vi "CTL_Level SpecV2.vi"(6 "Index(n-1) In":i32[](array[numeric]), 7 "Full Config 2":T1, 8 "error in (no error)":errorcluster, 9 "Level IN inches":dbl=8.853199052567236, 10 "Index B":i32=3, 11 "Index A":i32=3) -> (0 "error out":errorcluster, 2 "Enable":bool, 3 "Specs Out":T5, 4 "Index(n-1) Out":i32[](array[numeric]))   [LabVIEW 2024]
doc: "Determine the row index and Specification from the Config File Spec Table for the given level. \nAlso detemines the flag state for these Flags:\n Switch Zone = Resitor switch levels must occur in this zone\n R In Range Zone = Resistor value must be specified level\n R measure = When to take the measurement to record."
uses:
  Control Definitions/DEF_SpecsOut.ctl
  Control Definitions/Def PumpCtlRefs.ctl
  Control Definitions/Def FullCfg.ctl
  Control Definitions/Def BenchCfg.ctl
  Control Definitions/Def Bench Status.ctl
  Control Definitions/Ded LUT_Status.ctl
  Control Definitions/Ded Spec RNG.ctl
panel:
  out "Index(n)":i32
  out "Boolean":bool=TRUE
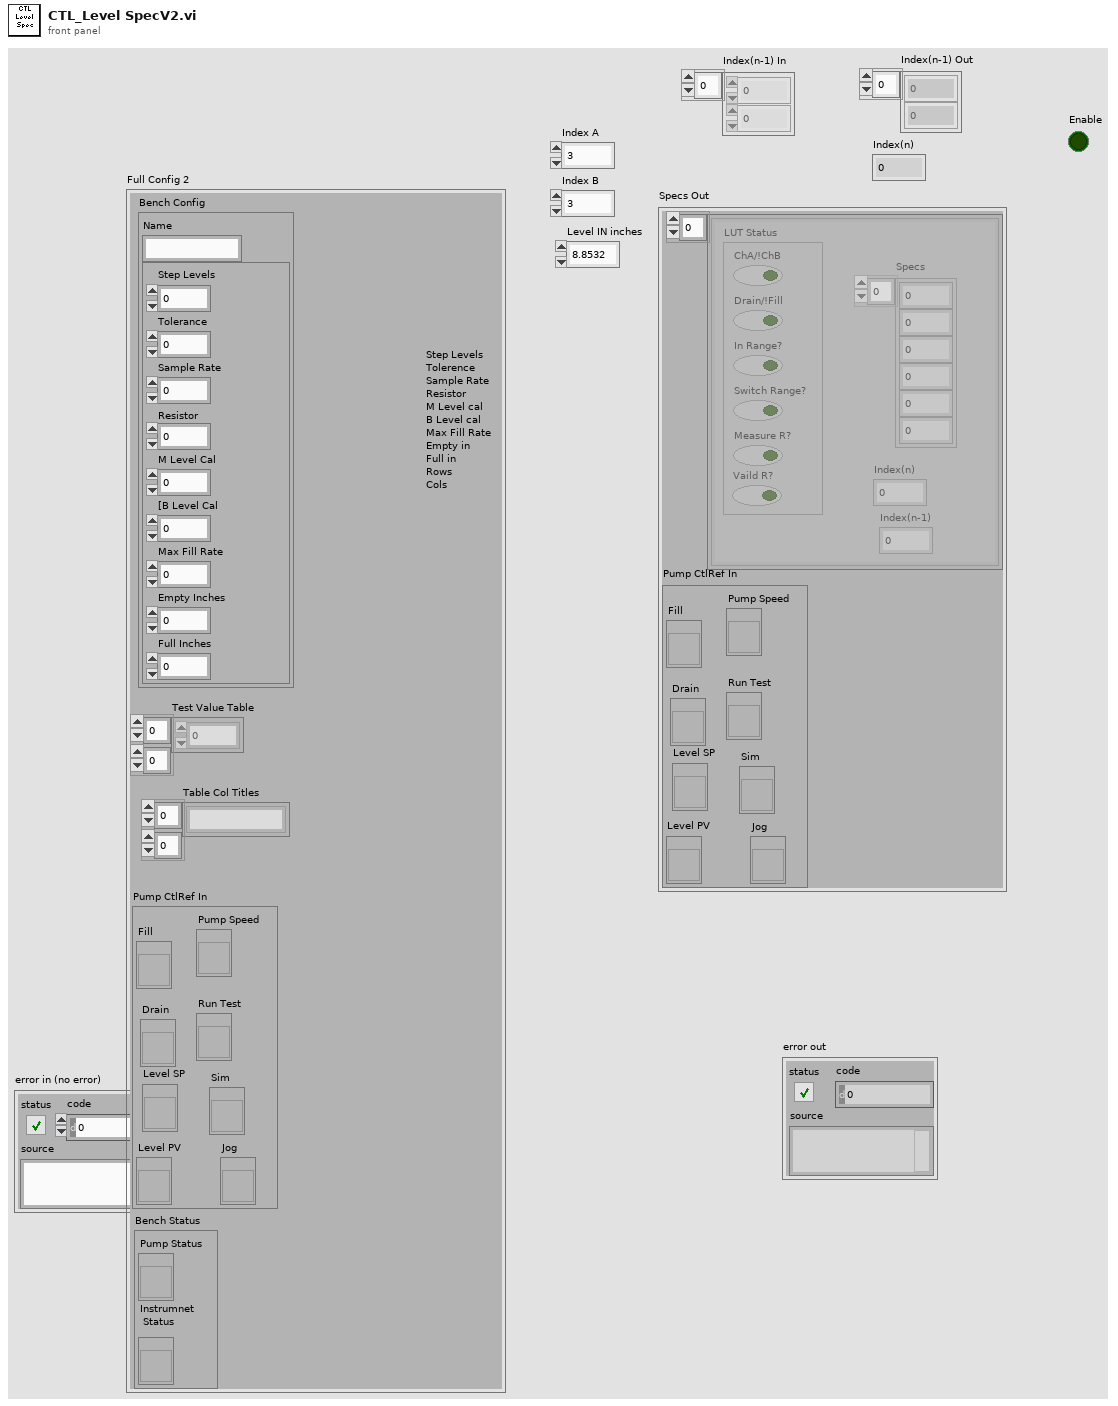
[diagram p1: front panel]
types:
  T1 = typedef "Def FullCfg.ctl" = cluster{"Bench Config":T2, "Test Value Table ":dbl[][], "Table Col Titles":string[][], "Pump CtlRef In":T3, "Bench Status":T4}
  T2 = typedef "Def BenchCfg.ctl" = cluster{"Name":string, cluster{"Step Levels":dbl, "Tolerance":dbl, "Sample Rate":dbl, "Resistor":dbl, "M Level Cal":dbl, "[B Level Cal":dbl, "Max Fill Rate":dbl, "Empty Inches":dbl, "Full Inches":dbl}}
  T3 = typedef "Def PumpCtlRefs.ctl" = cluster{"Fill ":refnum<vi>, "Drain":refnum<vi>, "Level PV":refnum<vi>, "Pump Speed":refnum<vi>, "Run Test":refnum<vi>, "Sim":refnum<vi>, "Jog":refnum<vi>, "Level SP":refnum<vi>}
  T4 = typedef "Def Bench Status.ctl" = cluster{"Pump Status":refnum<vi>, "Instrumnet\n Status":refnum<vi>}
  T5 = typedef "DEF_SpecsOut.ctl" = cluster{"aSpecsTable":T6[], "Pump CtlRef In":T3}
  T6 = typedef "Ded Spec RNG.ctl" = cluster{"Specs":dbl[], "Index(n)":i32, "LUT Status":T7, "Index(n-1)":i32}
  T7 = typedef "Ded LUT_Status.ctl" = cluster{"ChA/!ChB":bool, "Drain/!Fill":bool, "In Range?":bool, "Switch Range?":bool, "Measure R?":bool, "Vaild R?":bool}
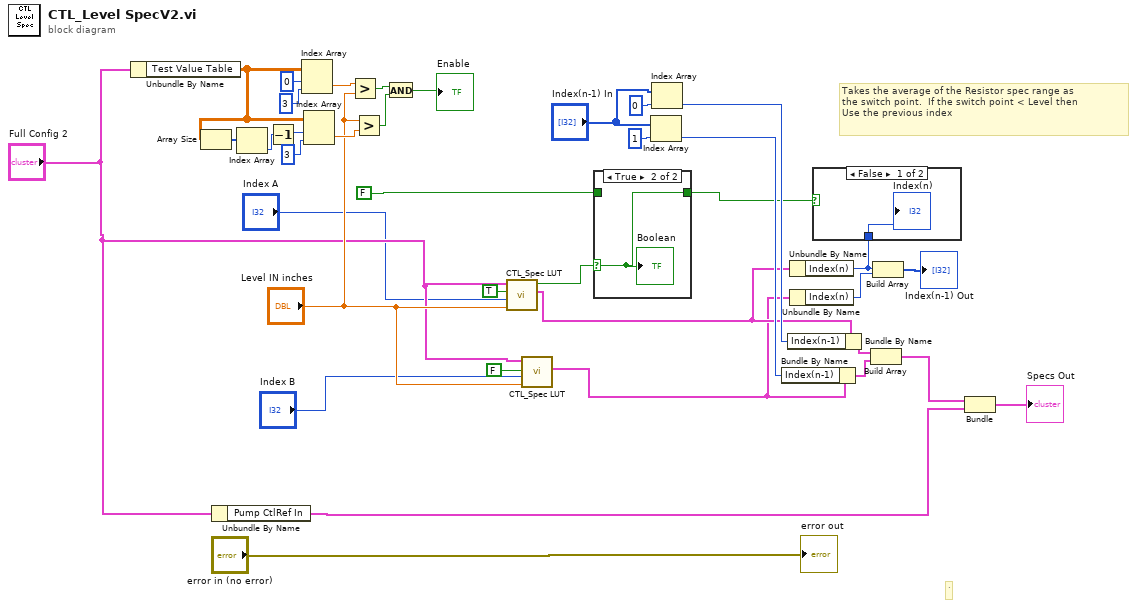
[diagram p0: block diagram]
diagram:
  # "`"
  # "Takes the average of the Resistor spec range as \nthe switch point.  If the switch point < Level then \nUse the previous index"
  n1 = Unbundle By Name("Full Config 2") -> ("Test Value Table"=w15:dbl[][])
  n2 = Array Size(array=w15) -> (size(s)=w13:i32[])
  n3 = Unbundle By Name("Full Config 2") -> ("Pump CtlRef In"=w5:T3)
  n4 = Index Array(array=w13) -> (element=w12:i32)  [unwired: 1 in]
  n5 = Decrement(x=w12) -> (x-1=w14:i32)
  n6 = Index Array(array=w15, index (row)=0, index (col)=3 ("disabled index (col)")) -> (element=w21:dbl)
  n7 = Index Array(array=w15, index (row)=w14, index (col)=3 ("disabled index (col)")) -> (element=w20:dbl)
  n8 = Greater?(x=w21, y="Level IN inches") -> (0:w17:bool)
  n9 = Greater?(x="Level IN inches", y=w20) -> (0:w18:bool)
  n10 = And(x=w17, y=w18) -> (x .and. y?=→"Enable":bool)
  n11 = call "CTL_Spec LUT.vi"("Level IN inches"="Level IN inches", "Index"="Index A", "ChA/!ChB"=TRUE, "Full Cfg"="Full Config 2") -> ("Spec RNG"=w2:T6, "In Range?"=w7:bool)  [unwired: 5 in, 1 out]
  n12 = call "CTL_Spec LUT.vi"("Level IN inches"="Level IN inches", "Index"="Index B", "ChA/!ChB"=FALSE, "Full Cfg"="Full Config 2") -> ("Spec RNG"=w1:T6)  [unwired: 5 in, 2 out]
  n13 = case shown="True" w7 {
    selector: w7 -> [_ w39]
    tunnel: [w38 w39] -> w25
    tunnel: FALSE -> [w38 _]
    frame False {
    }
    frame True {
      "Boolean" <- w39
    }
  }
  n14 = Index Array(array="Index(n-1) In", index=1) -> (element=w31:i32)
  n15 = Index Array(array="Index(n-1) In", index=0) -> (element=w30:i32)
  n16 = Bundle By Name(cluster=w1, "Index(n-1)"=w31) -> (w32:T6)
  n17 = Bundle By Name(cluster=w2, "Index(n-1)"=w30) -> (w33:T6)
  n18 = Unbundle By Name(w2) -> ("Index(n)"=w26:i32)
  n19 = Unbundle By Name(w1) -> ("Index(n)"=w29:i32)
  n20 = case shown="False" w25 {
    tunnel: w26 -> [w40 _]
    frame False {
      "Index(n)" <- w40
    }
    frame True {
    }
  }
  n21 = Build Array(w33, w32) -> (w11:T6[])
  n22 = Build Array(w26, w29) -> (→"Index(n-1) Out":i32[])
  n23 = Bundle(w11, "Pump CtlRef In"=w5) -> (→"Specs Out":cluster{T6[], "Pump CtlRef In":T3})  [unwired: 1 in]
  "error out" <- "error in (no error)"
